vi "怪物攻击.vi"() -> ()   [LabVIEW 2013]
panel:
  in  "停止":bool
  in  "怪兽 2":bool=TRUE
  in  "怪兽":bool
  in  "枚举":enum16{"初始化", "后退", "施法", "出击"}(ring)
  in  "13":bool
  in  "12":bool
  in  "11":bool
  in  "10":bool
  in  "9":bool
  in  "8":bool
  in  "7":bool
  in  "6":bool
  in  "5":bool
  in  "4":bool
  in  "3":bool
  in  "2":bool
  in  "1":bool
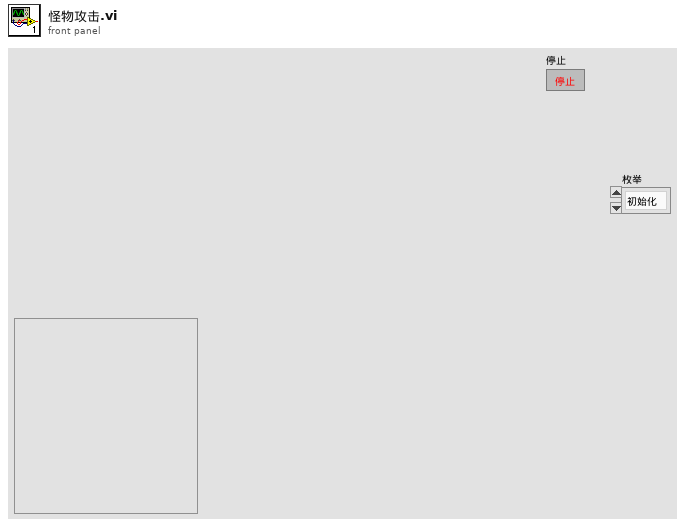
[diagram p1: front panel]
types:
  T1 = cluster{bool, bool, bool, bool, bool, bool, bool, bool, bool, bool, bool, bool, bool}
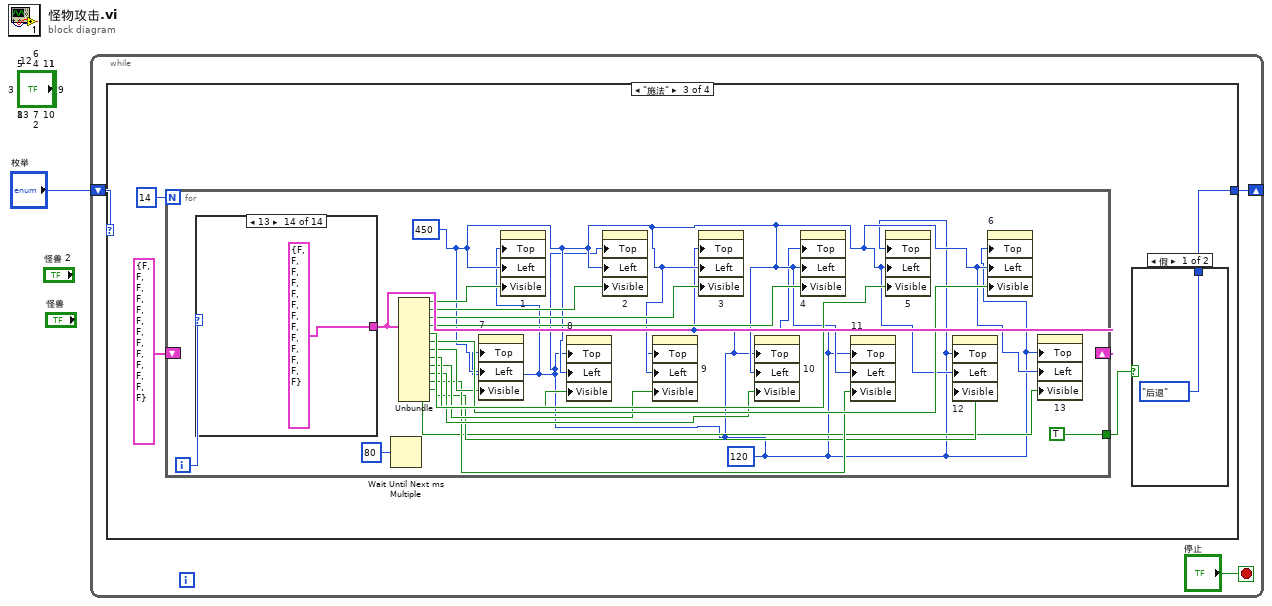
[diagram p0: block diagram]
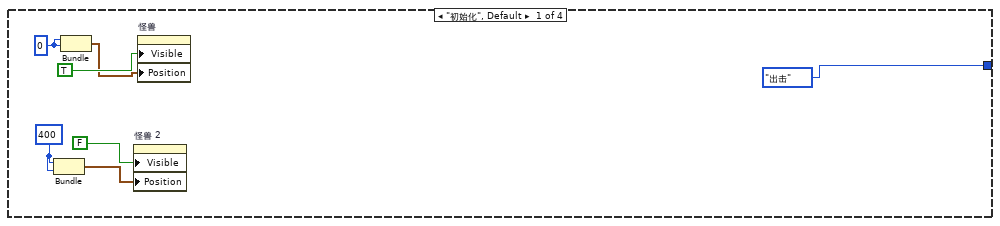
[diagram p2: hidden frame]
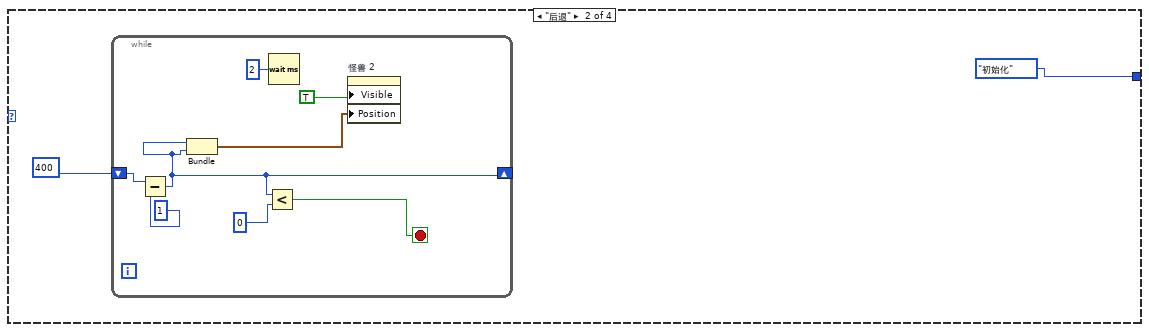
[diagram p3: hidden frame]
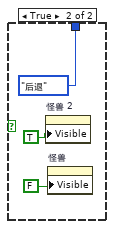
[diagram p4: hidden frame]
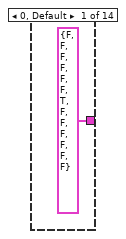
[diagram p5: hidden frame]
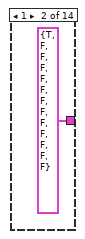
[diagram p6: hidden frame]
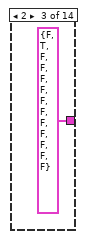
[diagram p7: hidden frame]
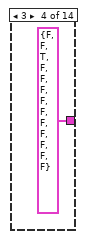
[diagram p8: hidden frame]
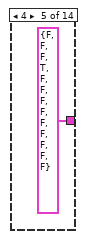
[diagram p9: hidden frame]
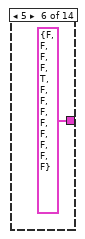
[diagram p10: hidden frame]
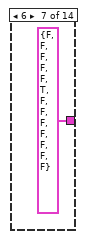
[diagram p11: hidden frame]
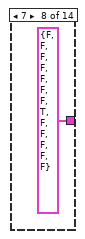
[diagram p12: hidden frame]
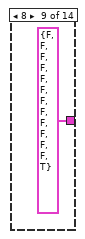
[diagram p13: hidden frame]
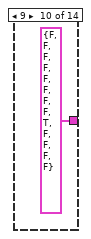
[diagram p14: hidden frame]
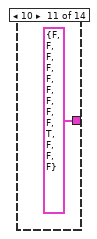
[diagram p15: hidden frame]
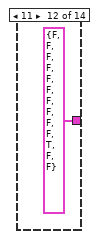
[diagram p16: hidden frame]
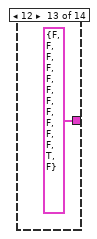
[diagram p17: hidden frame]
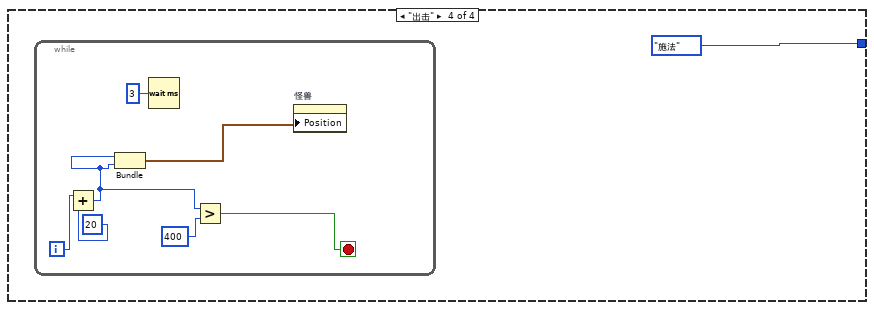
[diagram p18: hidden frame]
diagram:
  n1 = while {
    shift-right: [w3] -> _
    shift-left: "枚举" -> [w4]
    stop <- "停止" stop-if-true
    n2 = case shown="\"施法\"" w4 {
      tunnel: [enum16{"初始化", "后退", "施法", "出击"}."出击" ("枚举") enum16{"初始化", "后退", "施法", "出击"}."初始化" ("枚举") w22 enum16{"初始化", "后退", "施法", "出击"}."施法" ("枚举")] -> w3
      frame "初始化", Default {
        w10 = 400
        w11 = 0
        n3 = Bundle(w10, w10) -> (w6:cluster{i32, i32})  [unwired: 1 in]
        n4 = Bundle(w11, w11) -> (w7:cluster{i32, i32})  [unwired: 1 in]
        n5 = property on="怪兽 2" class="Bool"("Visible"=FALSE, "Position"=w6) -> ()  [unwired: 2 in, 2 out]
        n6 = property on="怪兽" class="Bool"("Visible"=TRUE, "Position"=w7) -> ()  [unwired: 2 in, 2 out]
      }
      frame "后退" {
        n7 = while {
          shift-right: [w16] -> _
          shift-left: 400 -> [w17]
          stop <- w18 stop-if-true
          n8 = Subtract(x=w17, y=1) -> (x-y=w16:i32)
          n9 = Bundle(w16, w16) -> (w14:cluster{i32, i32})  [unwired: 1 in]
          n10 = Less?(x=w16, y=0) -> (x < y?=w18:bool)
          n11 = Wait (ms)(milliseconds to wait=u32 2 ("等待时间（毫秒）")) -> ()  [unwired: 1 out]
          n12 = property on="怪兽 2" class="Bool"("Visible"=TRUE, "Position"=w14) -> ()  [unwired: 2 in, 2 out]
        }
      }
      frame "施法" {
        n13 = for {
          N: 14 -> [_]
          shift-right: [w47] -> _
          shift-left: T1 {FALSE, FALSE, FALSE, FALSE, FALSE, FALSE, FALSE, FALSE, FALSE, FALSE, FALSE, FALSE, FALSE} -> [_]
          tunnel: [TRUE] -> w23
          i -> [w48]
          w31 = 120
          w33 = 450
          n14 = case shown="13" w48 {
            tunnel: [T1 {FALSE, FALSE, FALSE, FALSE, FALSE, FALSE, TRUE, FALSE, FALSE, FALSE, FALSE, FALSE, FALSE} T1 {TRUE, FALSE, FALSE, FALSE, FALSE, FALSE, FALSE, FALSE, FALSE, FALSE, FALSE, FALSE, FALSE} T1 {FALSE, TRUE, FALSE, FALSE, FALSE, FALSE, FALSE, FALSE, FALSE, FALSE, FALSE, FALSE, FALSE} T1 {FALSE, FALSE, TRUE, FALSE, FALSE, FALSE, FALSE, FALSE, FALSE, FALSE, FALSE, FALSE, FALSE} T1 {FALSE, FALSE, FALSE, TRUE, FALSE, FALSE, FALSE, FALSE, FALSE, FALSE, FALSE, FALSE, FALSE} T1 {FALSE, FALSE, FALSE, FALSE, TRUE, FALSE, FALSE, FALSE, FALSE, FALSE, FALSE, FALSE, FALSE} T1 {FALSE, FALSE, FALSE, FALSE, FALSE, TRUE, FALSE, FALSE, FALSE, FALSE, FALSE, FALSE, FALSE} T1 {FALSE, FALSE, FALSE, FALSE, FALSE, FALSE, FALSE, TRUE, FALSE, FALSE, FALSE, FALSE, FALSE} T1 {FALSE, FALSE, FALSE, FALSE, FALSE, FALSE, FALSE, FALSE, FALSE, FALSE, FALSE, FALSE, TRUE} T1 {FALSE, FALSE, FALSE, FALSE, FALSE, FALSE, FALSE, FALSE, TRUE, FALSE, FALSE, FALSE, FALSE} T1 {FALSE, FALSE, FALSE, FALSE, FALSE, FALSE, FALSE, FALSE, FALSE, TRUE, FALSE, FALSE, FALSE} T1 {FALSE, FALSE, FALSE, FALSE, FALSE, FALSE, FALSE, FALSE, FALSE, FALSE, TRUE, FALSE, FALSE} T1 {FALSE, FALSE, FALSE, FALSE, FALSE, FALSE, FALSE, FALSE, FALSE, FALSE, FALSE, TRUE, FALSE} T1 {FALSE, FALSE, FALSE, FALSE, FALSE, FALSE, FALSE, FALSE, FALSE, FALSE, FALSE, FALSE, FALSE}] -> w47
            frame 0, Default {
            }
            frame 1 {
            }
            frame 2 {
            }
            frame 3 {
            }
            frame 4 {
            }
            frame 5 {
            }
            frame 6 {
            }
            frame 7 {
            }
            frame 8 {
            }
            frame 9 {
            }
            frame 10 {
            }
            frame 11 {
            }
            frame 12 {
            }
            frame 13 {
            }
          }
          n15 = Wait Until Next ms Multiple(millisecond multiple=u32 80 ("毫秒倍数")) -> ()  [unwired: 1 out]
          n16 = Unbundle(w47) -> (w46:bool, w45:bool, w44:bool, w43:bool, w42:bool, w41:bool, w40:bool, w39:bool, w38:bool, w37:bool, w36:bool, w35:bool, w34:bool)
          n17 = property on="7" class="Bool"("Top"=w31, "Left"=w33, "Visible"=w40) -> ()  [unwired: 2 in, 2 out]
          n18 = property on="1" class="Bool"("Top"=w31, "Left"=w33, "Visible"=w46) -> ()  [unwired: 2 in, 2 out]
          n19 = property on="8" class="Bool"("Top"=w31, "Left"=w33, "Visible"=w39) -> ()  [unwired: 2 in, 2 out]
          n20 = property on="2" class="Bool"("Top"=w31, "Left"=w33, "Visible"=w45) -> ()  [unwired: 2 in, 2 out]
          n21 = property on="9" class="Bool"("Top"=w31, "Left"=w33, "Visible"=w38) -> ()  [unwired: 2 in, 2 out]
          n22 = property on="3" class="Bool"("Top"=w31, "Left"=w33, "Visible"=w44) -> ()  [unwired: 2 in, 2 out]
          n23 = property on="10" class="Bool"("Top"=w31, "Left"=w33, "Visible"=w37) -> ()  [unwired: 2 in, 2 out]
          n24 = property on="4" class="Bool"("Top"=w31, "Left"=w33, "Visible"=w43) -> ()  [unwired: 2 in, 2 out]
          n25 = property on="11" class="Bool"("Top"=w31, "Left"=w33, "Visible"=w36) -> ()  [unwired: 2 in, 2 out]
          n26 = property on="5" class="Bool"("Top"=w31, "Left"=w33, "Visible"=w42) -> ()  [unwired: 2 in, 2 out]
          n27 = property on="12" class="Bool"("Top"=w31, "Left"=w33, "Visible"=w35) -> ()  [unwired: 2 in, 2 out]
          n28 = property on="6" class="Bool"("Top"=w31, "Left"=w33, "Visible"=w41) -> ()  [unwired: 2 in, 2 out]
          n29 = property on="13" class="Bool"("Top"=w31, "Left"=w33, "Visible"=w34) -> ()  [unwired: 2 in, 2 out]
        }
        n30 = case shown="假" w23 {
          tunnel: [enum16{"初始化", "后退", "施法", "出击"}."后退" ("枚举") enum16{"初始化", "后退", "施法", "出击"}."后退" ("枚举")] -> w22
          frame False {
          }
          frame True {
            n31 = property on="怪兽 2" class="Bool"("Visible"=TRUE) -> ()  [unwired: 2 in, 2 out]
            n32 = property on="怪兽" class="Bool"("Visible"=FALSE) -> ()  [unwired: 2 in, 2 out]
          }
        }
      }
      frame "出击" {
        n33 = while {
          i -> [w69]
          stop <- w64 stop-if-true
          n34 = Add(x=w69, y=20) -> (x+y=w67:i32)
          n35 = Bundle(w67, w67) -> (w65:cluster{i32, i32})  [unwired: 1 in]
          n36 = Wait (ms)(milliseconds to wait=u32 3 ("等待时间（毫秒）")) -> ()  [unwired: 1 out]
          n37 = Greater?(x=w67, y=400) -> (0:w64:bool)
          n38 = property on="怪兽" class="Bool"("Position"=w65) -> ()  [unwired: 2 in, 2 out]
        }
      }
    }
  }
